vi "Change Camera.vi"(8 "error in (no error)":errorcluster, 10 "New Camera":string, 11 "Camera Actor in":refnum<class "Camera Actor.lvclass">) -> (0 "error out":errorcluster, 3 "Camera Actor out":refnum<class "Camera Actor.lvclass">)   [LabVIEW 2020, in "Camera Actor.lvlib" / "Camera Actor.lvclass"]
uses:
  Camera Actor.lvclass
  Camera Actor.lvclass/Camera Actor.ctl
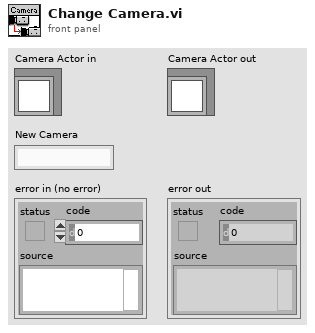
[diagram p1: front panel]
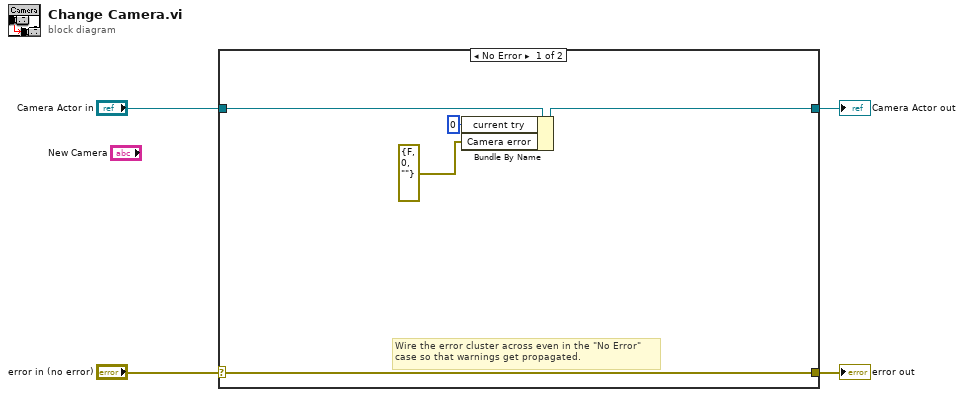
[diagram p0: block diagram]
diagram:
  n1 = case shown="No Error" "error in (no error)" {
    selector: "error in (no error)" -> [w8 w11]
    tunnel: [w8 w11] -> w3
    tunnel: [w7 w10] -> w1
    tunnel: "Camera Actor in" -> [w9 w10]
    frame No Error {
      # "Wire the error cluster across even in the \"No Error\"\ncase so that warnings get propagated."
      n2 = Bundle By Name(cluster=w9, "current try"=u8 0, "Camera error"=errorcluster {"status"=FALSE, "code"=0, "source"=""}) -> (w7:refnum<class "Camera Actor.lvclass">)
    }
    frame Error {
    }
  }
  "error out" <- w3
  "Camera Actor out" <- w1
